vi "CheckFile.vi"(8 "error in (no error)":errorcluster, 11 "path":path) -> (0 "error out":errorcluster, 3 "path out":path)   [LabVIEW 2024]
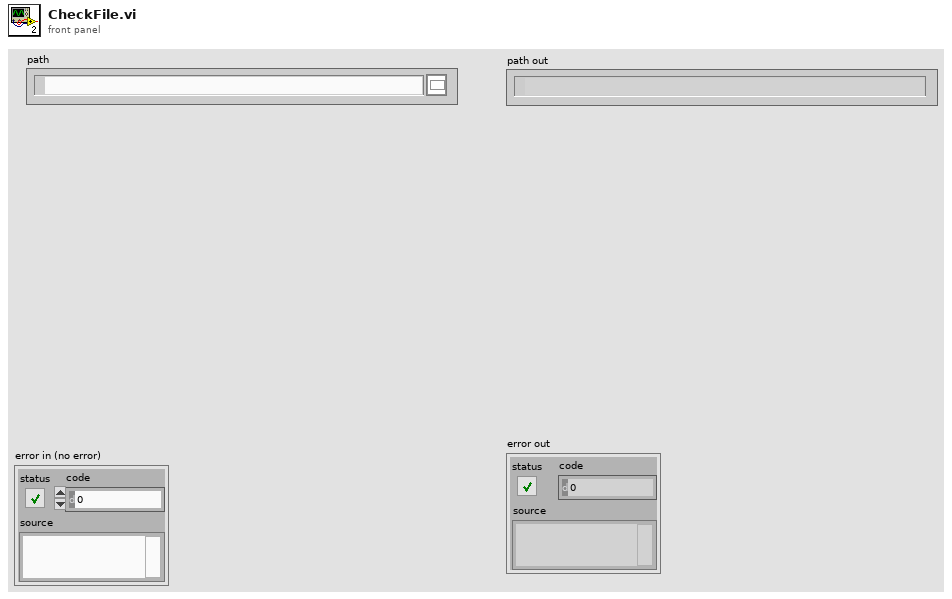
[diagram p1: front panel]
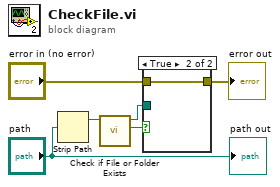
[diagram p0: block diagram]
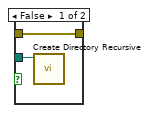
[diagram p2: hidden frame]
diagram:
  n1 = Strip Path(path="path") -> (stripped path=w6:path)  [unwired: 1 out]
  n2 = call <vilib>:"Check if File or Folder Exists.vi"("path"=w6) -> ("file or folder exists?"=w5:bool, "dup path"=w4:path)  [unwired: 8 in, 1 out]
  n3 = case shown="True" w5 {
    tunnel: w4 -> [w8 _]
    tunnel: "error in (no error)" -> [w7 w9]
    tunnel: [w7 w9] -> w2
    frame False {
      n4 = call <vilib>:"Create Directory Recursive.vi"("directory"=w8) -> ()  [unwired: 4 in, 3 out]
    }
    frame True {
    }
  }
  "error out" <- w2
  "path out" <- "path"
